vi "A_doThis.vi"(10 "input":dbl) -> (2 "output":dbl)   [LabVIEW 2016, in "LibA.lvlib"]
uses:
  LibA.lvlib
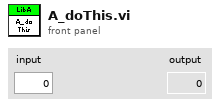
[diagram p1: front panel]
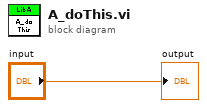
[diagram p0: block diagram]
diagram:
  "output" <- "input"
